vi "getVariablesToSet.vi"(11 "ActiveDev in":string) -> (2 "variables to set":string[](array[string]), 3 "ActiveDev out":string)   [LabVIEW 2011]
uses:
  C:/Program Files/National Instruments/LabVIEW 2011/resource/objmgr/daqmx.rc
panel:
  in  "error in (no error)":errorcluster
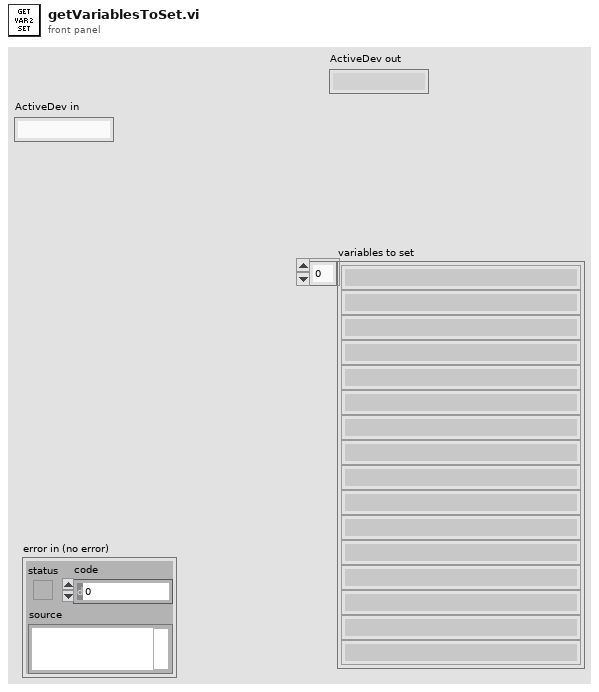
[diagram p1: front panel]
types:
  T1 = typedef "mysql_authentication.ctl" = cluster{"User":string, "Password":string, "Database":string}
  T2 = cluster{"Port":u16, "IP Address":string, "Authentication":T1}
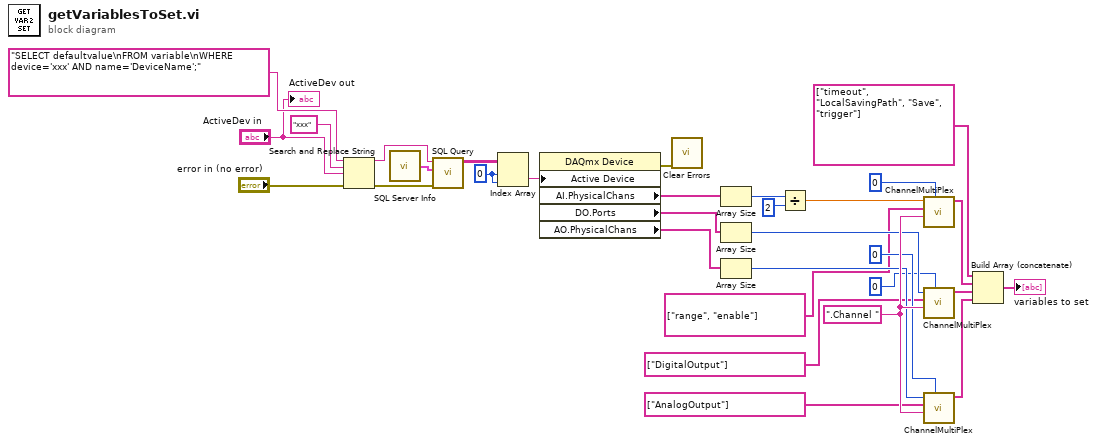
[diagram p0: block diagram]
diagram:
  w2 = 0 ("index (row)")
  w31 = ".Channel " ("string")
  n1 = Search and Replace String(input string="SELECT defaultvalue\nFROM variable\nWHERE  device='xxx' AND name='DeviceName';", search string="xxx", replace string="ActiveDev in", error in="error in (no error)") -> (result string=w8:string, error out=w9:errorcluster)  [unwired: 4 in, 2 out]
  n2 = call "SQL Server Info.vi"() -> ("SQL Server Info"=w5:T2)
  n3 = call "SQL Query.vi"("error in (no error)"=w9, "SQL Server Info"=w5, "Query"=w8) -> ("data"=w3:string[][])  [unwired: 7 in, 1 out]
  n4 = Index Array(array=w3, index (row)=w2, index (col)=w2) -> (element=w1:string)
  n5 = property class="DAQmx Device"("Active Device"=w1) -> (error out=w11:errorcluster, "AI.PhysicalChans"=w14:tag[], "DO.Ports"=w15:tag[], "AO.PhysicalChans"=w16:tag[])  [unwired: 2 in, 1 out]
  n6 = call "Clear Errors.vi"("error in (no error)"=w11) -> ()  [unwired: 6 in, 1 out]
  n7 = Array Size(array=w14) -> (size(s)=w12:i32)
  n8 = Array Size(array=w15) -> (size(s)=w21:i32)
  n9 = Array Size(array=w16) -> (size(s)=w25:i32)
  n10 = Divide(x=w12, y=2) -> (x/y=w19:dbl)
  n11 = call "ChannelMultiPlex.vi"("start"=0, "string"=w31, "set following Variables"=string[] ["range", "enable"], "Numeric"=w19) -> ("Array"=w26:string[])  [unwired: 6 in, 1 out]
  n12 = call "ChannelMultiPlex.vi"("start"=0, "string"=w31, "set following Variables"=string[] ["DigitalOutput"], "Numeric"=w21) -> ("Array"=w27:string[])  [unwired: 6 in, 1 out]
  n13 = call "ChannelMultiPlex.vi"("start"=0, "string"=w31, "set following Variables"=string[] ["AnalogOutput"], "Numeric"=w25) -> ("Array"=w28:string[])  [unwired: 6 in, 1 out]
  n14 = Build Array (concatenate)(string[] ["timeout", "LocalSavingPath", "Save", "trigger"] ("set following Variables"), w26, w27, w28) -> (→"variables to set":string[])
  "ActiveDev out" <- "ActiveDev in"
